vi "Read hWnd.vi"(8 "error in (no error)":errorcluster, 11 "LV MDI in":refnum<class "LV MDI.lvclass">) -> (0 "error out":errorcluster, 2 "hWnd":u64, 3 "LV MDI out":refnum<class "LV MDI.lvclass">)   [LabVIEW 2016]
uses:
  LV MDI.lvclass
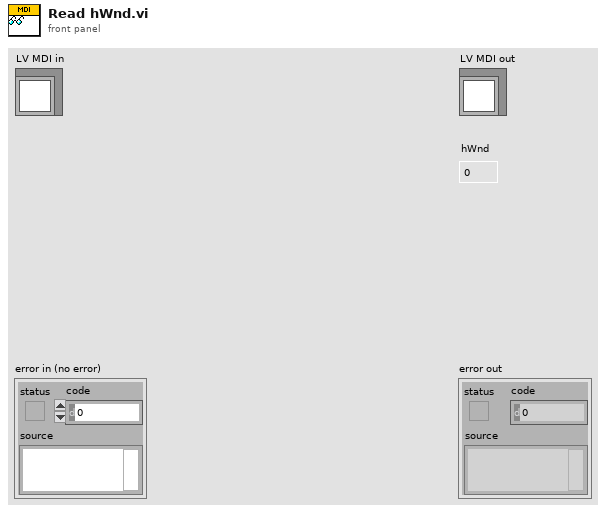
[diagram p1: front panel]
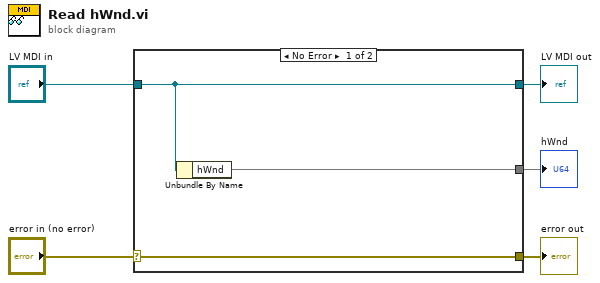
[diagram p0: block diagram]
diagram:
  n1 = case shown="No Error" "error in (no error)" {
    selector: "error in (no error)" -> [w8 w9]
    tunnel: [w8 w9] -> w4
    tunnel: [w7 w10] -> w2
    tunnel: "LV MDI in" -> [w7 w10]
    tunnel: [w6 _] -> w1
    frame No Error {
      n2 = Unbundle By Name(w7) -> ("hWnd"=w6)
    }
    frame Error {
    }
  }
  "error out" <- w4
  "LV MDI out" <- w2
  "hWnd" <- w1
